vi "SP Read From INI File.vi"(6 "Step Number":i32=1, 7 "De-Embed Data In":bool, 8 "error in (no error)":errorcluster, 9 "Display In":T1={"Lock Control"=FALSE, "Retain Settings"=TRUE, "Formatted Data"=FALSE, "Plot Orientation"=enum."Single", "Plot Controls"=[{"Trace Orientation"=enum."Overlay", "Frequency"={"Change Frequency"=FALSE, "Start"=500.0, "Stop"=1500.0, "Units"=enum."MHz"}, "Markers"=[], "Traces"=[]}, {"Trace Orientation"=enum."Overlay", "Frequency"={"Change Frequency"=FALSE, "Start"=500.0, "Stop"=1500.0, "Units"=enum."MHz"}, "Markers"=[], "Traces"=[]}, {"Trace Orientation"=enum."Overlay", "Frequency"={"Change Frequency"=FALSE, "Start"=500.0, "Stop"=1500.0, "Units"=enum."MHz"}, "Markers"=[], "Traces"=[]}, {"Trace Orientation"=enum."Overlay", "Frequency"={"Change Frequency"=FALSE, "Start"=500.0, "Stop"=1500.0, "Units"=enum."MHz"}, "Markers"=[], "Traces"=[]}]} {"Plot Controls"."Traces"."Reference" format="%#.2g"; "Plot Controls"."Traces"."Display Data" items=["Data", "Memory", "Data/Memory"]; "Plot Controls"."Traces"."Format" items=["Log Mag", "Phase", "Expanded Phase", "Delay", "Smith", "Polar", "Lin Mag", "SWR", "Loss", "Real", "Imaginary"]; "Plot Controls"."Traces"."Scale" min=0.001 step=1.0 format="%#.2g"; "Plot Controls"."Traces"."Position" min=0.0 max=10.0; "Plot Controls"."Frequency"."Stop" format="%.3g"; "Plot Controls"."Frequency"."Start" format="%.3g"}, 10 "Requested Stimulus In":T9={"Use Instrument Settings"=FALSE, "Blank Frequencies"=FALSE, "Sweep Type"=enum."Linear", "Sweep"={"Fstart"=500.0, "Fstop"=1500.0, "Units"=enum."MHz", "Points"=201}, "Power (dBm)"=999.0, "IFBW (Hz)"=-1.0, "Sweep Time (s)"=-1.0, "Calibration"={"State"=FALSE, "String"=""}} {"Sweep Time (s)" format="%.3g"}, 11 "Data to Read":enum16{"Calibration", "Display", "De-Embed"}(ring)) -> (0 "error out":errorcluster, 1 "Display Out":T1={"Lock Control"=FALSE, "Retain Settings"=TRUE, "Formatted Data"=FALSE, "Plot Orientation"=enum."Single", "Plot Controls"=[{"Trace Orientation"=enum."Overlay", "Frequency"={"Change Frequency"=FALSE, "Start"=500.0, "Stop"=1500.0, "Units"=enum."MHz"}, "Markers"=[], "Traces"=[]}, {"Trace Orientation"=enum."Overlay", "Frequency"={"Change Frequency"=FALSE, "Start"=500.0, "Stop"=1500.0, "Units"=enum."MHz"}, "Markers"=[], "Traces"=[]}, {"Trace Orientation"=enum."Overlay", "Frequency"={"Change Frequency"=FALSE, "Start"=500.0, "Stop"=1500.0, "Units"=enum."MHz"}, "Markers"=[], "Traces"=[]}, {"Trace Orientation"=enum."Overlay", "Frequency"={"Change Frequency"=FALSE, "Start"=500.0, "Stop"=1500.0, "Units"=enum."MHz"}, "Markers"=[], "Traces"=[]}]} {"Plot Controls"."Traces"."Reference" format="%#.2g"; "Plot Controls"."Traces"."Display Data" items=["Data", "Memory", "Data/Memory"]; "Plot Controls"."Traces"."Format" items=["Log Mag", "Phase", "Expanded Phase", "Delay", "Smith", "Polar", "Lin Mag", "SWR", "Loss", "Real", "Imaginary"]; "Plot Controls"."Traces"."Scale" min=0.001 step=1.0 format="%#.2g"; "Plot Controls"."Traces"."Position" min=0.0 max=10.0; "Plot Controls"."Frequency"."Stop" format="%.3g"; "Plot Controls"."Frequency"."Start" format="%.3g"}, 2 "Requested Stimulus Out":T9={"Use Instrument Settings"=FALSE, "Blank Frequencies"=FALSE, "Sweep Type"=enum."Linear", "Sweep"={"Fstart"=500.0, "Fstop"=1500.0, "Units"=enum."MHz", "Points"=201}, "Power (dBm)"=999.0, "IFBW (Hz)"=-1.0, "Sweep Time (s)"=-1.0, "Calibration"={"State"=FALSE, "String"=""}} {"Sweep Time (s)" format="%.3g"}, 3 "Requested Cal State":T10, 4 "Exists?":bool, 5 "De-Embed Data Out":bool)   [LabVIEW 2011]
uses:
  TypeDefs/SP Calibration State.ctl
  TypeDefs/SP Stimulus Parameters.ctl
  TypeDefs/SP Frequency Units.ctl
  TypeDefs/SP Display Parameters.ctl
  TypeDefs/SP Display Plot Controls Cluster.ctl
  TypeDefs/SP Marker Cluster.ctl
  TypeDefs/SP Marker Type.ctl
  TypeDefs/SP Display Trace Controls.ctl
  TypeDefs/SP Display Format.ctl
  TypeDefs/SP Display Data.ctl
  <vilib>/Utility/config.llb/Read Key (String).vi
  <vilib>/Utility/config.llb/NI_LVConfig.lvlib
panel:
  # "Div"
  # "Div"
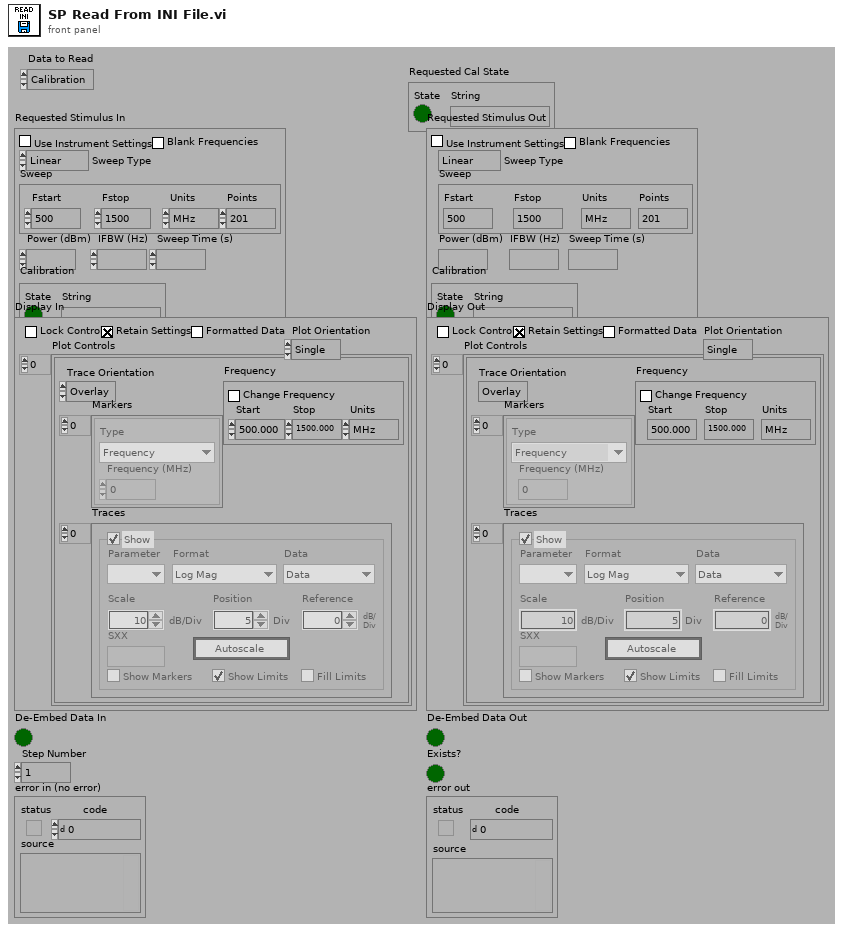
[diagram p1: front panel]
types:
  T1 = typedef "SP Display Parameters.ctl" = cluster{"Lock Control":bool, "Retain Settings":bool, "Formatted Data":bool, "Plot Orientation":enum32{"Single", "Dual", "Quad"}, "Plot Controls":T2[]}
  T2 = typedef "SP Display Plot Controls Cluster.ctl" = cluster{"Trace Orientation":enum32{"Overlay", "Split"}, "Frequency":cluster{"Change Frequency":bool, "Start":dbl, "Stop":dbl, "Units":T3}, "Markers":T4[], "Traces":T6[]}
  T3 = typedef "SP Frequency Units.ctl" = enum16{"Hz", "kHz", "MHz", "GHz", "Points"}
  T4 = typedef "SP Marker Cluster.ctl" = cluster{"Type":T5, "Frequency (MHz)":dbl}
  T5 = typedef "SP Marker Type.ctl" = enum16{"Frequency", "Trace Maximum", "Trace Minimum", "Limit Maximum", "Limit Minimum"}
  T6 = typedef "SP Display Trace Controls.ctl" = cluster{"Trace On":bool, "Measure":i32, "Format":T7, "Autoscale":bool, "Reference":dbl, "\nRefUnit":string, "Position":dbl, "Scale":dbl, "ScaleUnit":string, "LimitOn":bool, "LimitFill":bool, "Display Data":T8, "Show Markers":bool, "SXX":string}
  T7 = typedef "SP Display Format.ctl" = i32
  T8 = typedef "SP Display Data.ctl" = u16
  T9 = typedef "SP Stimulus Parameters.ctl" = cluster{"Use Instrument Settings":bool, "Blank Frequencies":bool, "Sweep Type":enum32{"Linear", "Logarithmic", "List", "Power", "CW"}, "Sweep":cluster{"Fstart":dbl, "Fstop":dbl, "Units":T3, "Points":i32}, "Power (dBm)":dbl, "IFBW (Hz)":dbl, "Sweep Time (s)":dbl, "Calibration":T10}
  T10 = typedef "SP Calibration State.ctl" = cluster{"State":bool, "String":string}
  T11 = typedef "NI_LVConfig.lvlib/Config Data RefNum.ctl" = refnum<k1>
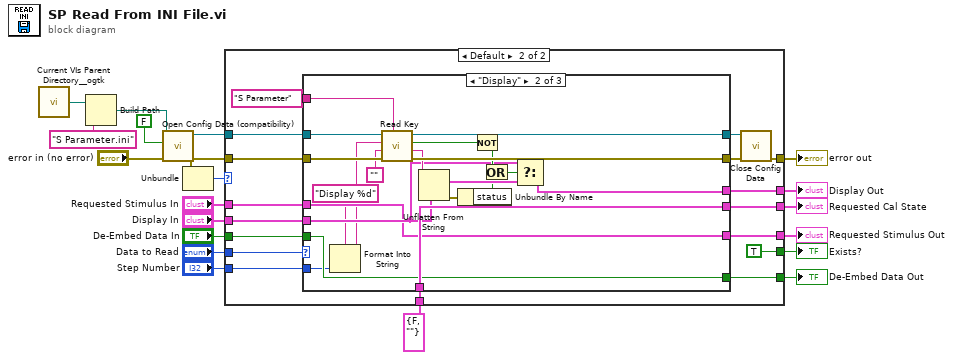
[diagram p0: block diagram]
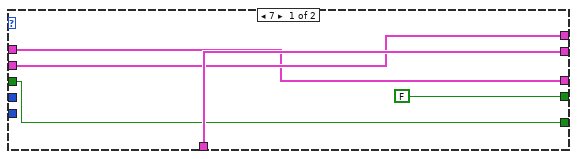
[diagram p2: hidden frame]
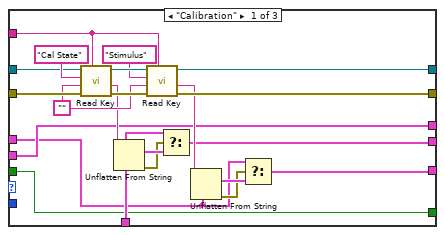
[diagram p3: hidden frame]
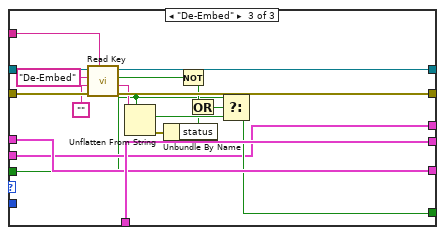
[diagram p4: hidden frame]
diagram:
  n1 = call "Current VIs Parent Directory__ogtk.vi"() -> ("Parent Directory (+ Relative)"=w1:path)  [unwired: 5 in]
  n2 = Build Path(base path=w1, name or relative path="S Parameter.ini") -> (appended path=w17:path)
  n3 = call <vilib>:"Open Config Data (compatibility).vi"("error in (no error)"="error in (no error)", "create file if necessary (T)"=FALSE ("create file if necessary? (T)"), "configuration file path"=w17) -> ("error out"=w11:errorcluster, "refnum"=w16:T11)  [unwired: 6 in, 1 out]
  n4 = Unbundle(w11) -> ("code"=w10:i32)  [unwired: 2 out]
  n5 = case shown="Default" w10 {
    tunnel: [_ w42] -> w19
    tunnel: w11 -> [_ w39]
    tunnel: w16 -> [_ w38]
    tunnel: "Data to Read" -> [_ w37]
    tunnel: [w25 w35] -> w14
    tunnel: [w22 w34] -> w13
    tunnel: [w23 w33] -> w12
    tunnel: T10 {"State"=FALSE, "String"=""} ("Requested Cal State") -> [w25 w32]
    tunnel: [FALSE ("Exists?") TRUE ("Exists?")] -> w8
    tunnel: "Display In" -> [w23 w30]
    tunnel: "Requested Stimulus In" -> [w22 w29]
    tunnel: "De-Embed Data In" -> [w21 w28]
    tunnel: [w21 w27] -> w3
    tunnel: "Step Number" -> [_ w26]
    frame 7 {
    }
    frame Default {
      n6 = case shown="\"Display\"" w37 {
        tunnel: [w62 w81 w100] -> w41
        tunnel: [w61 w82 w101] -> w40
        tunnel: w39 -> [w58 w85 w104]
        tunnel: w38 -> [w57 w84 w103]
        tunnel: "S Parameter" ("section") -> [w56 w83 w102]
        tunnel: w32 -> [w48 w80 w99]
        tunnel: [w49 w80 w99] -> w35
        tunnel: [w51 w69 w89] -> w34
        tunnel: [w45 w76 w87] -> w33
        tunnel: w30 -> [w45 w70 w87]
        tunnel: w29 -> [w44 w69 w89]
        tunnel: w28 -> [w43 w68 w86]
        tunnel: [w43 w68 w88] -> w27
        tunnel: w26 -> [_ w67 _]
        frame "Calibration" {
          w55 = ""
          n7 = call-poly <vilib>:"Read Key.vi"("section"=w56, "error in (no error)"=w58, "default value"=w55, "key"="Cal State" ("section"), "refnum"=w57) -> ("error out"=w63:errorcluster, "value"=w54:string, "refnum out"=w64:T11)  [unwired: 1 in, 3 out]
          n8 = Unflatten From String(type=w48, binary string=w54) -> (value=w50:T10, error out=w47:errorcluster)  [unwired: 1 in, 3 out]
          n9 = call-poly <vilib>:"Read Key.vi"("section"=w56, "error in (no error)"=w63, "default value"=w55, "key"="Stimulus", "refnum"=w64) -> ("error out"=w61:errorcluster, "value"=w53:string, "refnum out"=w62:T11)  [unwired: 1 in, 3 out]
          n10 = Select(t=w48, s=w47, f=w50) -> (s? t:f=w49:T10)
          n11 = Unflatten From String(type=w44, binary string=w53) -> (value=w52:T9, error out=w46:errorcluster)  [unwired: 1 in, 3 out]
          n12 = Select(t=w44, s=w46, f=w52) -> (s? t:f=w51:T9)
        }
        frame "Display" {
          n13 = Format Into String(format string="Display %d" ("section"), w67) -> (resulting string=w65:string)  [unwired: 2 in, 1 out]
          n14 = call-poly <vilib>:"Read Key.vi"("section"=w83, "error in (no error)"=w85, "default value"="", "key"=w65, "refnum"=w84) -> ("error out"=w82:errorcluster, "value"=w78:string, "found?"=w75:bool, "refnum out"=w81:T11)  [unwired: 1 in, 2 out]
          n15 = Unflatten From String(type=w70, binary string=w78) -> (value=w77:T1, error out=w72:errorcluster)  [unwired: 1 in, 3 out]
          n16 = Unbundle By Name(w72) -> ("status"=w73:bool)
          n17 = Not(x=w75) -> (.not. x?=w74:bool)
          n18 = Or(x=w74, y=w73) -> (x .or. y?=w71:bool)
          n19 = Select(t=w70, s=w71, f=w77) -> (s? t:f=w76:T1)
        }
        frame "De-Embed" {
          n20 = call-poly <vilib>:"Read Key.vi"("section"=w102, "error in (no error)"=w104, "default value"="", "key"="De-Embed" ("section"), "refnum"=w103) -> ("error out"=w101:errorcluster, "value"=w97:string, "found?"=w94:bool, "refnum out"=w100:T11)  [unwired: 1 in, 2 out]
          n21 = Unflatten From String(type=w86, binary string=w97) -> (value=w95:bool, error out=w91:errorcluster)  [unwired: 1 in, 3 out]
          n22 = Unbundle By Name(w91) -> ("status"=w92:bool)
          n23 = Not(x=w94) -> (.not. x?=w93:bool)
          n24 = Or(x=w93, y=w92) -> (x .or. y?=w90:bool)
          n25 = Select(t=w86, s=w90, f=w95) -> (s? t:f=w88:bool)
        }
      }
      n26 = call <vilib>:"Close Config Data.vi"("error in (no error)"=w40, "refnum"=w41) -> ("error out"=w42:errorcluster)  [unwired: 1 in, 8 out]
    }
  }
  "error out" <- w19
  "Display Out" <- w12
  "Requested Cal State" <- w14
  "Requested Stimulus Out" <- w13
  "Exists?" <- w8
  "De-Embed Data Out" <- w3
